vi "UART Init.vi"(9 "pConfig":T1, 10 "Channel":u8, 11 "DevHandle":i32) -> (1 "pConfig out":T1, 3 "function return":i32)   [LabVIEW 2010, in "usb2uart.lvlib"]
doc: "int WINAPI UART_Init(int DevHandle, unsigned char Channel, PUART_CONFIG pConfig);"
uses:
  usb2uart.lvlib
  USB2XXX.dll
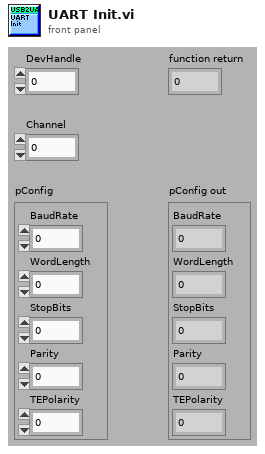
[diagram p1: front panel]
types:
  T1 = cluster{"BaudRate":u32, "WordLength":u8, "StopBits":u8, "Parity":u8, "TEPolarity":u8}
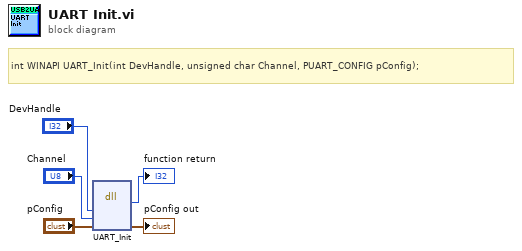
[diagram p0: block diagram]
diagram:
  # "int WINAPI UART_Init(int DevHandle, unsigned char Channel, PUART_CONFIG pConfig);"
  n1 = dll-call lib="E:/OtherWork/STM32/USB2XXX_Example/trunk/Labview/PublicFiles/USB2XXX.*" fn="UART_Init"("DevHandle"="DevHandle", "Channel"="Channel", "pConfig"="pConfig") -> (→"function return":i32, "pConfig"=→"pConfig out":T1)  [unwired: 5 in, 2 out]
